vi "ql2_token_build.vi"(10 "term":string, 11 "token in (0:random)":u64 format="%016x") -> (3 "message":string)   [LabVIEW 2017, in "rethinkdb.lvlib"]
uses:
  rethinkdb.lvlib
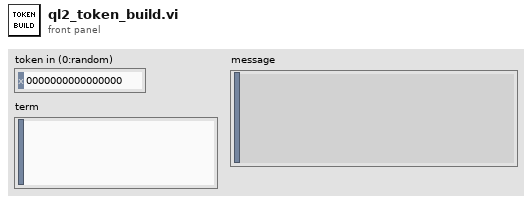
[diagram p1: front panel]
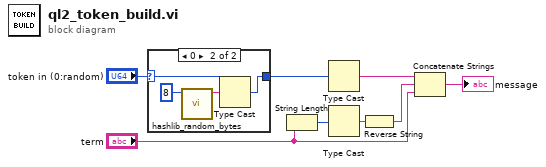
[diagram p0: block diagram]
diagram:
  n1 = case shown="0" "token in (0:random)" {
    selector: "token in (0:random)" -> [w9 w11]
    tunnel: [w9 w10] -> w3
    frame Default {
    }
    frame 0 {
      n2 = call "hashlib_random_bytes.vi"("length (18bytes)"=8 ("length")) -> ("random bytes"=w12:string)  [unwired: 10 in]
      n3 = Type Cast(type=w11, x=w12) -> (*(type *) &x=w10:u64)
    }
  }
  n4 = String Length(string="term") -> (length=w5:i32)
  n5 = Type Cast(x=w3) -> (*(type *) &x=w7:string)  [unwired: 1 in]
  n6 = Type Cast(x=w5) -> (*(type *) &x=w6:string)  [unwired: 1 in]
  n7 = Reverse String(1:w6) -> (0:w8:string)
  n8 = Concatenate Strings(w7, w8, "term") -> (→"message":string)
